vi "PID Baustein IAG.vi"(0 "setpoint":sgl format="%.2f", 1 "output range":cluster{"output high":sgl, "output low":sgl}={"output high"=100.0, "output low"=-100.0} {"output low" format="%.2f"; "output high" format="%.2f"}, 2 "auto? (T)":bool=TRUE, 3 "manual control":sgl format="%.2f", 5 "process variable":sgl format="%.2f", 9 "PID gains":T3={"proportional gain (Kc)"=1.0, "integral time (Ti, min)"=0.01, "derivative time (Td, min)"=0.0} {"derivative time (Td, min)" format="%.3f"; "integral time (Ti, min)" format="%.3f"; "proportional gain (Kc)" format="%.3f"}, 11 "dt (s)":sgl=-1.0 format="%.3f", 12 "reinitialize? (F)":bool, 13 "Regler erzwingen":T1, 14 "Regler Interne Werte":sgl[](array[numeric])) -> (4 "output":sgl format="%.2f", 8 "Regler Werte":T2, 15 "dt out (s)":sgl format="%.3f")   [LabVIEW 2020, in "Regler.lvlib" / "Druckregler.lvlib"]
uses:
  Druckregler.lvlib
  Regler Interne Werte.ctl
  Regler Werte erzwingen.ctl
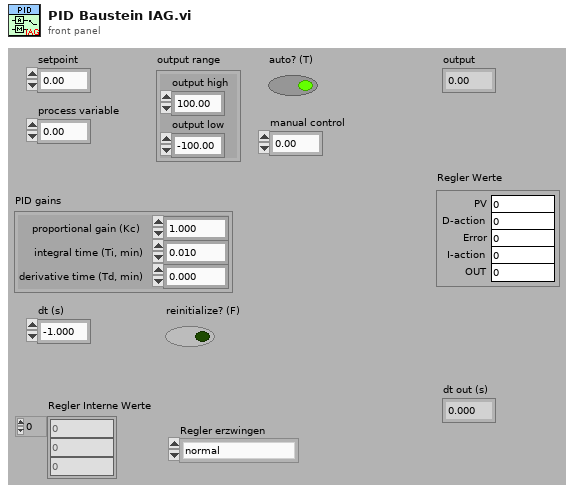
[diagram p1: front panel]
types:
  T1 = typedef "Regler.lvlib/Druckregler.lvlib/Regler Werte erzwingen.ctl" = enum16{"normal", "erzwingen"}
  T2 = typedef "Regler.lvlib/Druckregler.lvlib/Regler Interne Werte.ctl" = cluster{"PV":sgl, "D-action":sgl, "Error":sgl, "I-action":sgl, "OUT":sgl}
  T3 = cluster{"proportional gain (Kc)":sgl, "integral time (Ti, min)":sgl, "derivative time (Td, min)":sgl}
  T4 = cluster{"process variable":sgl, sgl, sgl, "Numerisch":sgl, "Numerisch":sgl}
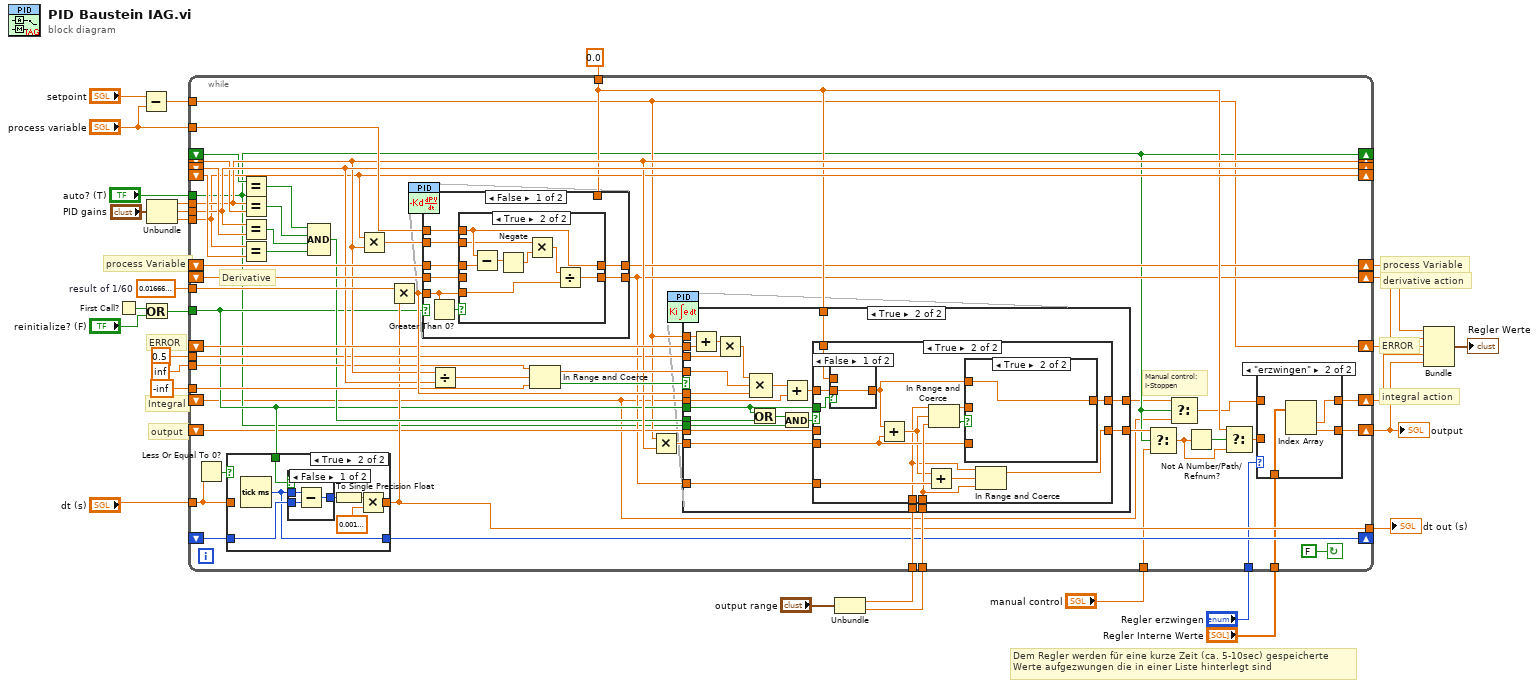
[diagram p0: block diagram]
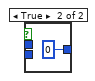
[diagram p4: hidden frame]
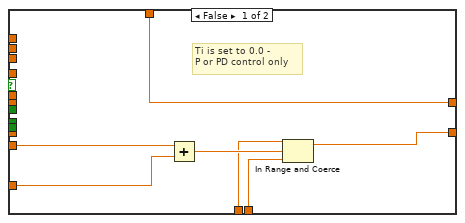
[diagram p5: hidden frame]
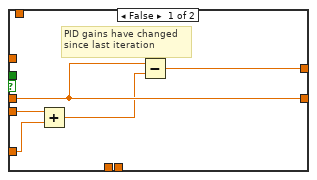
[diagram p6: hidden frame]
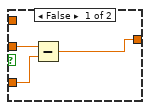
[diagram p7: hidden frame]
diagram:
  w15 = sgl 0.016666668  # result of 1/60
  # "Dem Regler werden für eine kurze Zeit (ca. 5-10sec) gespeicherte \nWerte aufgezwungen die in einer Liste hinterlegt sind"
  # "integral action"
  # "derivative action"
  # "process Variable"
  # "Integral"
  # "output"
  # "process Variable"
  # "ERROR"
  # "ERROR"
  n1 = First Call?() -> (First Call?: T/F=w29:bool)
  n2 = Subtract(x="setpoint", y="process variable") -> (x-y=w9:sgl)
  n3 = Or(x=w29, y="reinitialize? (F)") -> (x .or. y?=w19:bool)
  n4 = Unbundle("PID gains") -> ("proportional gain (Kc)"=w27:sgl, "integral time (Ti, min)"=w26:sgl, "derivative time (Td, min)"=w25:sgl)
  n5 = Unbundle("output range") -> ("output high"=w22:sgl, "output low"=w21:sgl)
  n6 = while {
    tunnel: w19 -> [w44]
    shift-left: _ -> [w56]
    shift-right: [w57] -> _
    shift-right: [w63] -> _
    shift-left: _ -> [w64]
    shift-right: [w65] -> _
    shift-left: _ -> [w81]
    shift-right: [w58] -> _
    shift-left: _ -> [w82]
    tunnel: w27 -> [w63]
    tunnel: w26 -> [w65]
    tunnel: w25 -> [w58]
    tunnel: "dt (s)" -> [w55]
    tunnel: w22 -> [w77]
    tunnel: w21 -> [w76]
    tunnel: "process variable" -> [w75]
    shift-right: [w39] -> w8
    shift-left: _ -> [w74]
    shift-right: [w38] -> w7
    shift-left: _ -> [w70]
    shift-right: [w40] -> w4
    shift-left: _ -> [w43]
    shift-right: [w37] -> w6
    shift-left: _ -> [w73]
    shift-right: [w42] -> w5
    shift-left: _ -> [w31]
    tunnel: w15 -> [w67]
    tunnel: sgl 0.5 ("y") -> [w62]
    tunnel: sgl inf ("upper limit") -> [w60]
    tunnel: sgl -inf ("lower limit") -> [w61]
    tunnel: sgl 0.0 -> [w45]
    shift-right: [w34] -> _
    shift-left: _ -> [w53]
    tunnel: "auto? (T)" -> [w34]
    tunnel: [w50] -> w13
    tunnel: "manual control" -> [w46]
    tunnel: w9 -> [w37]
    tunnel: "Regler erzwingen" -> [w36]
    tunnel: "Regler Interne Werte" -> [w35]
    stop <- FALSE continue-if-true
    # "Manual control:\nI-Stoppen"
    # "Derivative"
    n7 = Less Or Equal To 0?(x=w55) -> (x <= 0?=w54:bool)
    n8 = case shown="True" w54 {
      tunnel: [w90 w94] -> w50
      tunnel: w56 -> [w89 w93]
      tunnel: [w89 w92] -> w57
      tunnel: w55 -> [w90 _]
      tunnel: w44 -> [_ w91]
      frame False {
      }
      frame True {
        n9 = Tick Count (ms)() -> (millisecond timer value=w92:u32)
        n10 = case shown="False" w91 {
          tunnel: [w100 u32 0] -> w96
          tunnel: w93 -> [w99 _]
          tunnel: w92 -> [w98 _]
          frame False {
            n11 = Subtract(x=w98, y=w99) -> (x-y=w100:u32)
          }
          frame True {
          }
        }
        n12 = To Single Precision Float(number=w96) -> (single precision float=w95:sgl)
        n13 = Multiply(x=w95, y=sgl 0.001) -> (x*y=w94:sgl)
      }
    }
    n14 = Equal?(x=w53, y=w34) -> (x = y?=w51:bool)
    n15 = Equal?(x=w63, y=w64) -> (x = y?=w79:bool)
    n16 = Equal?(x=w65, y=w81) -> (x = y?=w78:bool)
    n17 = Equal?(x=w58, y=w82) -> (x = y?=w80:bool)
    n18 = Compound Arithmetic op=AND(w51, w79, w78, w80) -> (w52:bool)
    n19 = Multiply(x=w58, y=w63) -> (x*y=w69:sgl)
    n20 = Multiply(x=w67, y=w50) -> (x*y=w83:sgl)
    n21 = case shown="False" w44 {
      tunnel: w74 -> [w164 _]
      tunnel: w69 -> [w161 _]
      tunnel: w75 -> [w163 w176]
      tunnel: [w160 w176] -> w39
      tunnel: [w162 w175] -> w38
      tunnel: w70 -> [w158 _]
      tunnel: w83 -> [w157 _]
      tunnel: w45 -> [_ w175]
      frame False {
        n22 = Greater Than 0?(x=w157) -> (x > 0?=w159:bool)
        n23 = case shown="True" w159 {
          tunnel: w164 -> [w166 w172]
          tunnel: w157 -> [_ w171]
          tunnel: w163 -> [_ w169]
          tunnel: [w165 w170] -> w162
          tunnel: w161 -> [_ w167]
          tunnel: [w166 w169] -> w160
          tunnel: w158 -> [w165 _]
          frame False {
            # "dt = 0 min"
          }
          frame True {
            n24 = Subtract(x=w169, y=w172) -> (x-y=w174:sgl)
            n25 = Negate(x=w174) -> (-x=w168:sgl)
            n26 = Multiply(x=w167, y=w168) -> (x*y=w173:sgl)
            n27 = Divide(x=w173, y=w171) -> (x/y=w170:sgl)
          }
        }
      }
      frame True {
      }
    }
    n28 = Divide(x=w63, y=w65) -> (x/y=w68:sgl)
    n29 = In Range and Coerce(upper limit=w60, x=w68, lower limit=w61) -> (coerced(x)=w72:sgl, In Range?=w71:bool)
    n30 = Multiply(x=w37, y=w63) -> (x*y=w66:sgl)
    n31 = case shown="True" w71 {
      tunnel: w37 -> [_ w130]
      tunnel: w73 -> [_ w131]
      tunnel: w31 -> [_ w126]
      tunnel: [w102 w122] -> w33
      tunnel: w72 -> [_ w120]
      tunnel: w66 -> [w107 w124]
      tunnel: [w108 w121] -> w47
      tunnel: w43 -> [_ w123]
      tunnel: w38 -> [w106 w119]
      tunnel: w44 -> [_ w118]
      tunnel: w52 -> [_ w117]
      tunnel: w83 -> [_ w116]
      tunnel: w77 -> [w104 w114]
      tunnel: w76 -> [w103 w115]
      tunnel: w62 -> [_ w113]
      tunnel: w45 -> [w102 w112]
      tunnel: w34 -> [_ w109]
      frame False {
        # "Ti is set to 0.0 -\nP or PD control only"
        n32 = Add(x=w107, y=w106) -> (x+y=w105:sgl)
        n33 = In Range and Coerce(upper limit=w104, x=w105, lower limit=w103) -> (coerced(x)=w108:sgl)  [unwired: 1 out]
      }
      frame True {
        n34 = Add(x=w130, y=w131) -> (x+y=w129:sgl)
        n35 = Multiply(x=w129, y=w113) -> (x*y=w128:sgl)
        n36 = Compound Arithmetic op=MULTIPLY(w128, w120, w116) -> (w127:sgl)
        n37 = Or(x=w118, y=w117) -> (x .or. y?=w110:bool)
        n38 = Add(x=w127, y=w126) -> (x+y=w125:sgl)
        n39 = And(x=w110, y=w109) -> (x .and. y?=w111:bool)
        n40 = case shown="True" w111 {
          tunnel: w125 -> [_ w144]
          tunnel: w124 -> [w134 w140]
          tunnel: w123 -> [w136 _]
          tunnel: w118 -> [_ w146]
          tunnel: [w135 w142] -> w122
          tunnel: [w136 w149] -> w121
          tunnel: w119 -> [w133 w148]
          tunnel: w115 -> [_ w147]
          tunnel: w114 -> [_ w138]
          tunnel: w112 -> [_ w145]
          frame False {
            # "PID gains have changed\nsince last iteration"
            n41 = Add(x=w134, y=w133) -> (x+y=w132:sgl)
            n42 = Subtract(x=w136, y=w132) -> (x-y=w135:sgl)
          }
          frame True {
            n43 = case shown="False" w146 {
              tunnel: w145 -> [_ w156]
              tunnel: [w155 w156] -> w143
              tunnel: w144 -> [w155 _]
              frame False {
              }
              frame True {
              }
            }
            n44 = Add(x=w143, y=w140) -> (x+y=w139:sgl)
            n45 = Add(x=w139, y=w148) -> (x+y=w150:sgl)
            n46 = In Range and Coerce(upper limit=w138, x=w139, lower limit=w147) -> (coerced(x)=w137:sgl, In Range?=w141:bool)
            n47 = case shown="True" w141 {
              tunnel: w143 -> [_ w154]
              tunnel: [w151 w154] -> w142
              tunnel: w137 -> [w153 _]
              tunnel: w140 -> [w152 _]
              frame False {
                n48 = Subtract(x=w153, y=w152) -> (x-y=w151:sgl)
              }
              frame True {
              }
            }
            n49 = In Range and Coerce(upper limit=w138, x=w150, lower limit=w147) -> (coerced(x)=w149:sgl)  [unwired: 1 out]
          }
        }
      }
    }
    n50 = Select(t=w47, s=w34, f=w46) -> (s? t:f=w49:sgl)
    n51 = Select(t=w33, s=w34, f=w31) -> (s? t:f=w32:sgl)
    n52 = Not A Number/Path/Refnum?(number/path/refnum=w49) -> (NaN/Path/Refnum?=w48:bool)
    n53 = Select(t=w45, s=w48, f=w49) -> (s? t:f=w41:sgl)
    n54 = case shown="\"erzwingen\"" w36 {
      tunnel: w32 -> [w85 _]
      tunnel: [w85 w87] -> w42
      tunnel: w41 -> [w84 _]
      tunnel: [w84 w88] -> w40
      tunnel: w35 -> [_ w86]
      frame "normal", Default {
      }
      frame "erzwingen" {
        n55 = Index Array(array=w86) -> (element #1=w87:sgl, element #2=w88:sgl)  [unwired: 2 in]
      }
    }
  }
  "dt out (s)" <- w13
  "output" <- w4
  n56 = Bundle("process variable"=w8, w7, w6, "Numerisch"=w5, "Numerisch"=w4) -> (→"Regler Werte":T4)  [unwired: 1 in]
